vi "Ramp.vi"(3 "LoopPeriod":u64=1 caption="Loop Period (ms)", 4 "HoldTime":u64=1000 caption="Hold Time (ms)", 5 "RampTime":u64=1000 caption="Ramp Time (ms)", 6 "Mode":enum16{"Run", "Reset"}(ring), 7 "LoopCount":u64) -> (0 "Value":dbl, 1 "Outcome":enum16{"RampUp", "Hold", "RampDown", "Finished"}(ring))   [LabVIEW 2011]
panel:
  out "HoldCount":dbl=1.0
  in  "BaseCount":u64
  out "RampCount":dbl=1.0
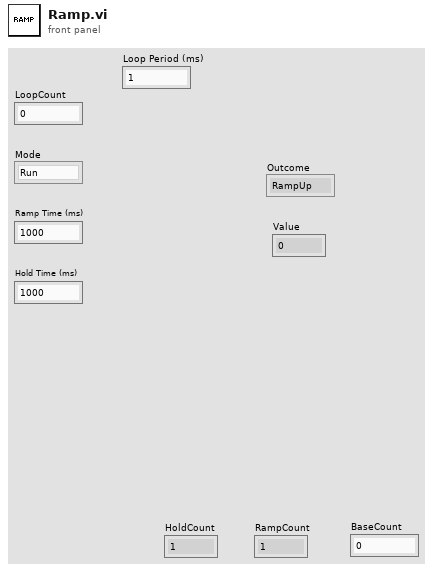
[diagram p1: front panel]
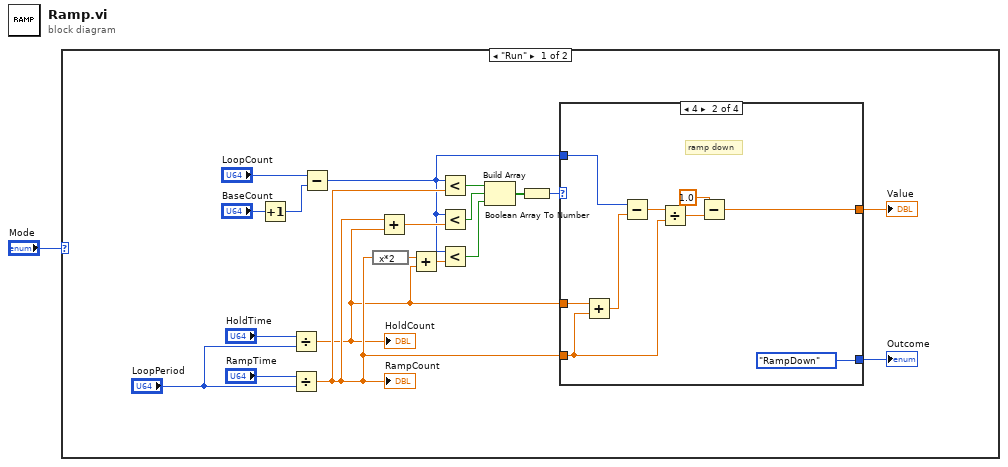
[diagram p0: block diagram]
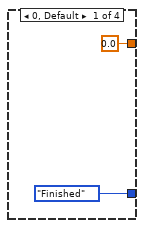
[diagram p2: hidden frame]
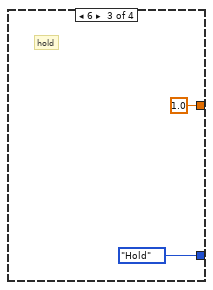
[diagram p3: hidden frame]
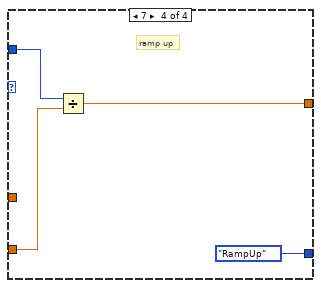
[diagram p4: hidden frame]
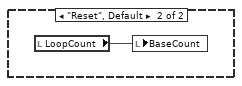
[diagram p5: hidden frame]
diagram:
  n1 = case shown="\"Run\"" "Mode" {
    frame "Run" {
      n2 = Increment(x="BaseCount") -> (x+1=w18:u64)
      n3 = Divide(x="HoldTime", y="LoopPeriod") -> (x/y=w3:dbl)
      "HoldCount" <- w3
      n4 = Divide(x="RampTime", y="LoopPeriod") -> (x/y=w4:dbl)
      "RampCount" <- w4
      n5 = Subtract(x="LoopCount", y=w18) -> (x-y=w2:u64)
      n6 = expression code="x*2"(w4) -> (w5:dbl)
      n7 = Add(x=w4, y=w3) -> (x+y=w14:dbl)
      n8 = Add(x=w5, y=w3) -> (x+y=w7:dbl)
      n9 = Less?(x=w2, y=w4) -> (x < y?=w13:bool)
      n10 = Less?(x=w2, y=w14) -> (x < y?=w12:bool)
      n11 = Less?(x=w2, y=w7) -> (x < y?=w6:bool)
      n12 = Build Array(w13, w12, w6) -> (w11:bool[])
      n13 = Boolean Array To Number(Boolean array=w11) -> (number=w10:u32)
      n14 = case shown="4" w10 {
        tunnel: [enum16{"RampUp", "Hold", "RampDown", "Finished"}."Finished" ("Outcome") enum16{"RampUp", "Hold", "RampDown", "Finished"}."RampDown" ("Outcome") enum16{"RampUp", "Hold", "RampDown", "Finished"}."Hold" ("Outcome") enum16{"RampUp", "Hold", "RampDown", "Finished"}."RampUp" ("Outcome")] -> w9
        tunnel: w4 -> [_ w27 _ w36]
        tunnel: w2 -> [_ w31 _ w37]
        tunnel: w3 -> [_ w30 _ _]
        tunnel: [0.0 ("Value") w24 1.0 ("Value") w35] -> w8
        frame 0, Default {
        }
        frame 4 {
          # "ramp down"
          n15 = Add(x=w30, y=w27) -> (x+y=w29:dbl)
          n16 = Subtract(x=w31, y=w29) -> (x-y=w28:dbl)
          n17 = Divide(x=w28, y=w27) -> (x/y=w26:dbl)
          n18 = Subtract(x=1.0, y=w26) -> (x-y=w24:dbl)
        }
        frame 6 {
          # "hold"
        }
        frame 7 {
          # "ramp up"
          n19 = Divide(x=w37, y=w36) -> (x/y=w35:dbl)
        }
      }
      "Outcome" <- w9
      "Value" <- w8
    }
    frame "Reset", Default {
      n20 = local read "LoopCount"() -> (w38:u64)
      n21 = local write "BaseCount"(w38) -> ()
    }
  }
